vi "Load Calc (SubVI).vi"(6 "process parameters in":T1, 9 "Leak load":dbl, 10 "HV-101":bool, 11 "Process load":dbl) -> (3 "process parameters out":T1)   [LabVIEW 2025]
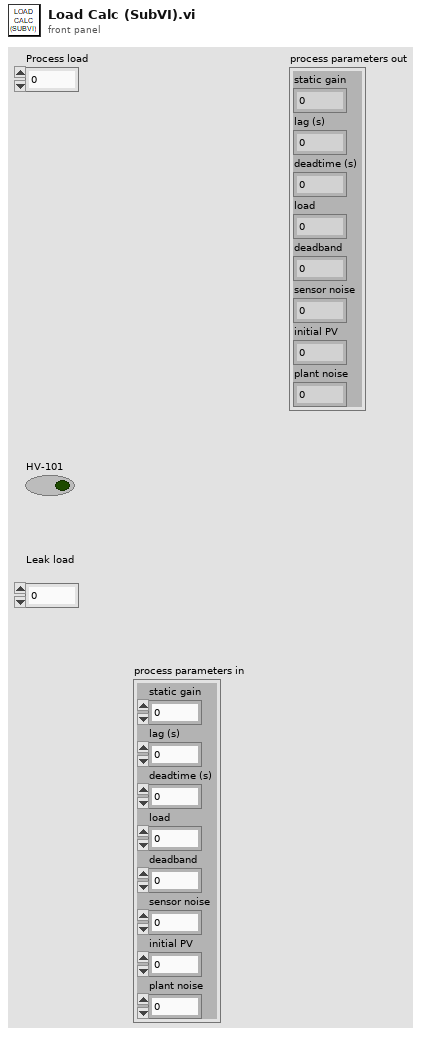
[diagram p1: front panel]
types:
  T1 = cluster{"static gain":dbl, "lag (s)":dbl, "deadtime (s)":dbl, "load":dbl, "deadband":dbl, "sensor noise":dbl, "initial PV":dbl, "plant noise":dbl}
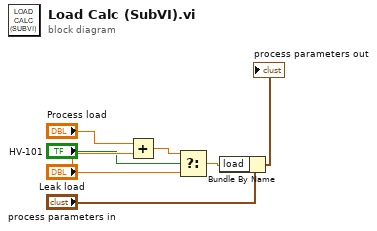
[diagram p0: block diagram]
diagram:
  n1 = Add(x="Process load", y="Leak load") -> (x+y=w3:dbl)
  n2 = Select(t=w3, s="HV-101", f="Leak load") -> (s? t:f=w1:dbl)
  n3 = Bundle By Name(cluster="process parameters in", "load"=w1) -> (→"process parameters out":T1)
